vi "KepcoDCPwr Initiate [TRG].vi"(0 "VISA Session":refnum<visa-resource-name>, 5 "Model In":string, 7 "channel name (\"\")":string="\"\"", 9 "Initiate Type":enum16{"Immediate", "Continuous"}(ring), 11 "error in (no error)":errorcluster {"code" format="%.0x"}, 12 "Continuous On/Off":bool) -> (4 "VISA Session Out":refnum<visa-resource-name>, 6 "Model Out":string, 8 "channel name out (\"\")":string="\"\"" caption="channel name Out (\"\")", 15 "error out":errorcluster {"code" format="%.0x"})   [LabVIEW 2010]
doc: "This VI initiates output changes that you previously specified.\n\nIf the power supply is not currently waiting for a trigger, the power supply waits for the trigger you specify with the KepcoDCPwr Configure Trigger Source.vi after you call this VI. After the power supply detects the trigger, it updates its voltage level and current limit to the values you specify with the KepcoDCPwr Configure Triggered Voltage Level.vi and KepcoDCPwr Configure Triggered Current Limit.vi VIs.\n\n\nIf the power supply is already waiting for a trigger, this VI does nothing and returns VI_SUCCESS."
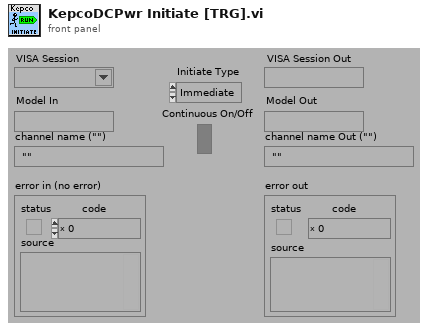
[diagram p1: front panel]
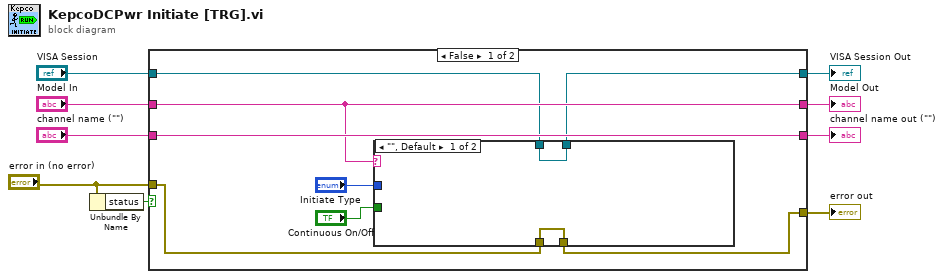
[diagram p0: block diagram]
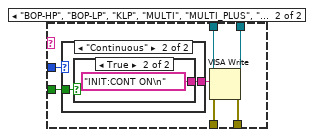
[diagram p2: hidden frame]
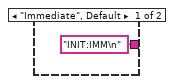
[diagram p3: hidden frame]
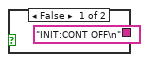
[diagram p4: hidden frame]
diagram:
  n1 = Unbundle By Name("error in (no error)") -> ("status"=w8:bool)
  n2 = case shown="False" w8 {
    tunnel: [w13 w35] -> w9
    tunnel: "error in (no error)" -> [w12 w35]
    tunnel: [w14 w34] -> w1
    tunnel: "VISA Session" -> [w15 w34]
    tunnel: [w16 w33] -> w2
    tunnel: "Model In" -> [w16 w33]
    tunnel: [w17 w32] -> w3
    tunnel: "channel name (\"\")" -> [w17 w32]
    frame False {
      n3 = case shown="\"\", Default" w16 {
        tunnel: w12 -> [w18 w25]
        tunnel: w15 -> [w19 w24]
        tunnel: [w19 w23] -> w14
        tunnel: [w18 w22] -> w13
        tunnel: "Initiate Type" -> [_ w21]
        tunnel: "Continuous On/Off" -> [_ w20]
        frame "", Default {
        }
        frame "BOP-HP", "BOP-LP", "KLP", "MULTI", "MULTI_PLUS", "STANDARD" {
          n4 = case shown="\"Continuous\"" w21 {
            tunnel: ["INIT:IMM\n" w28] -> w26
            tunnel: w20 -> [_ w29]
            frame "Immediate", Default {
            }
            frame "Continuous" {
              n5 = case shown="True" w29 {
                tunnel: ["INIT:CONT OFF\n" "INIT:CONT ON\n"] -> w28
                frame False {
                }
                frame True {
                }
              }
            }
          }
          n6 = VISA Write(VISA resource name=w24, write buffer=w26, error in (no error)=w25) -> (VISA resource name out=w23:refnum<visa-resource-name>, error out=w22:errorcluster)  [unwired: 1 out]
        }
      }
    }
    frame True {
    }
  }
  "error out" <- w9
  "Model Out" <- w2
  "channel name out (\"\")" <- w3
  "VISA Session Out" <- w1
